vi "myMaxAPDs.vi"(1 "Array":dbl[](array[numeric])) -> (0 "myMax":dbl)   [LabVIEW 2019]
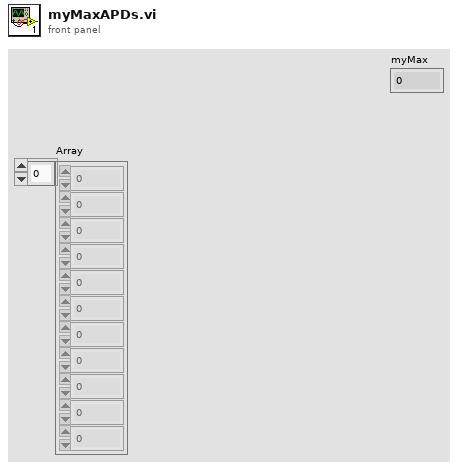
[diagram p1: front panel]
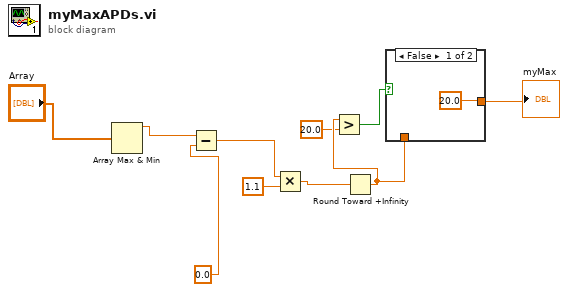
[diagram p0: block diagram]
diagram:
  n1 = Array Max & Min(array="Array") -> (max value=w3:dbl)  [unwired: 3 out]
  n2 = Subtract(x=w3, y=0.0) -> (x-y=w4:dbl)
  n3 = Multiply(x=w4, y=1.1) -> (x*y=w6:dbl)
  n4 = Round Toward +Infinity(x=w6) -> (ceil(x): smallest int >= x=w9:dbl)
  n5 = Greater?(x=w9, y=20.0) -> (0:w8:bool)
  n6 = case shown="False" w8 {
    tunnel: w9 -> [_ w12]
    tunnel: [20.0 w12] -> w10
    frame False {
    }
    frame True {
    }
  }
  "myMax" <- w10
